vi "_INIT_HalfCOS_LUT_16384.vi"() -> (0 "Init Data Out":fxp<+/-,16,14>[](array[numeric]))   [LabVIEW 2018]
panel:
  # "For Initialization VI requirements and help, please read directions located on Block Diagram."
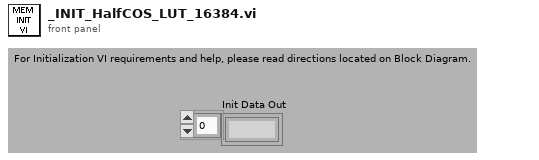
[diagram p1: front panel]
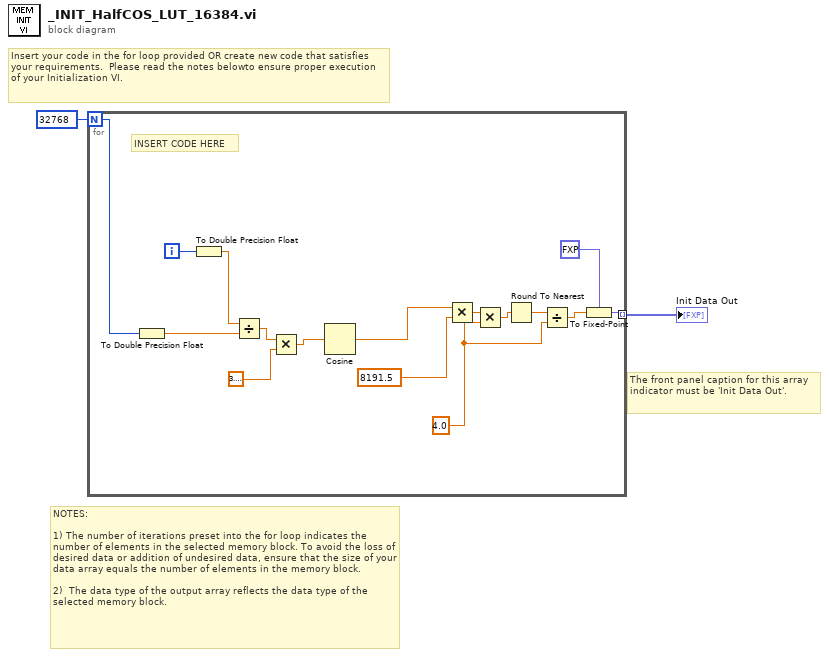
[diagram p0: block diagram]
diagram:
  # "The front panel caption for this array indicator must be 'Init Data Out'."
  # "NOTES:\n\n1) The number of iterations preset into the for loop indicates the number of elements in the selected memory block. To avoid the loss of desired data or addition of undesired data, ensure that the size of your data array equals the number of elements in the memory block.\n\n2)  The data type of the output array reflects the data type of the selected memory block."
  # "Insert your code in the for loop provided OR create new code that satisfies your requirements.  Please read the notes belowto ensure proper execution of your Initialization VI."
  n1 = for {
    N: 32768 ("Number of Elements") -> [w16]
    tunnel: [w10] -> w1 mode=indexing
    i -> [w18]
    w4 = 4.0 ("y")
    # "INSERT CODE HERE"
    n2 = To Double Precision Float(number=w16) -> (double precision float=w15:dbl)
    n3 = To Double Precision Float(number=w18) -> (double precision float=w17:dbl)
    n4 = Divide(x=w17, y=w15) -> (x/y=w14:dbl)
    n5 = Multiply(x=w14, y=3.141592653589793) -> (x*y=w12:dbl)
    n6 = Cosine(x=w12) -> (cos(x)=w3:dbl)
    n7 = Multiply(x=w3, y=8191.5) -> (x*y=w9:dbl)
    n8 = Multiply(x=w9, y=w4) -> (x*y=w6:dbl)
    n9 = Round To Nearest(number=w6) -> (nearest integer value=w7:dbl)
    n10 = Divide(x=w7, y=w4) -> (x/y=w5:dbl)
    n11 = To Fixed-Point(fixed-point type=fxp<+/-,16,14> 0.0, number=w5) -> (fixed-point=w10:fxp<+/-,16,14>)
  }
  "Init Data Out" <- w1
